vi "windowIcon.vi"(8 "Error In":errorcluster, 11 "LQGuiEngine In":refnum<class "LQGuiEngine.lvclass">) -> (0 "Error Out":errorcluster, 2 "Value":refnum<class "QIcon.lvclass">, 3 "LQGuiEngine Out":refnum<class "LQGuiEngine.lvclass">)   [LabVIEW 2014, in "LQGuiEngine.lvclass"]
doc: "LabVIEW-specific documentation is not yet available. See <b>http://doc.qt.io/qt-5/QGuiApplication.html#windowIcon</b>"
uses:
  LQGuiEngine.lvclass
  QIcon/QIcon.lvclass
  LQ Core/LQIdentity/LQIdentity.lvclass/LQIdentity.ctl
  LQ Core/LQSerialData/LQSerialData.lvclass/LQSerialData.ctl
  LQ Core/LQ Core.lvlib
  LQ Core/LQIdentity/LQIdentity.lvclass
  LQ Core/LQSerialData/LQSerialData.lvclass
panel:
  # "Copyright (c) 2016 Sze Howe Koh\n\nThis Source Code Form is subject to the terms of the Mozilla Public\nLicense, v. 2.0. If a copy of the MPL was not distributed with this\nfile, You can obtain one at http://mozilla.org/MPL/2.0/."
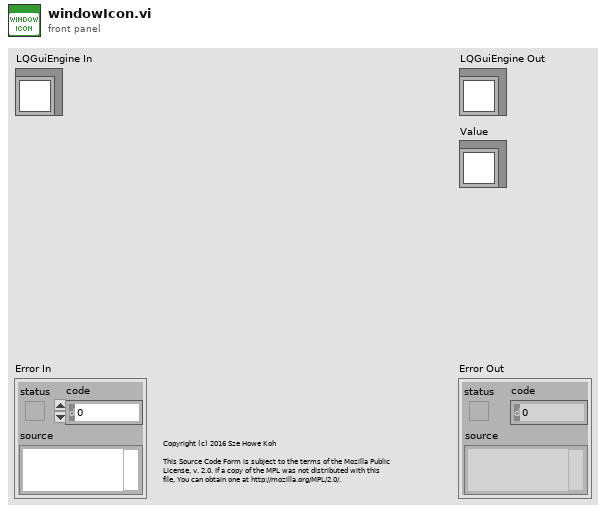
[diagram p1: front panel]
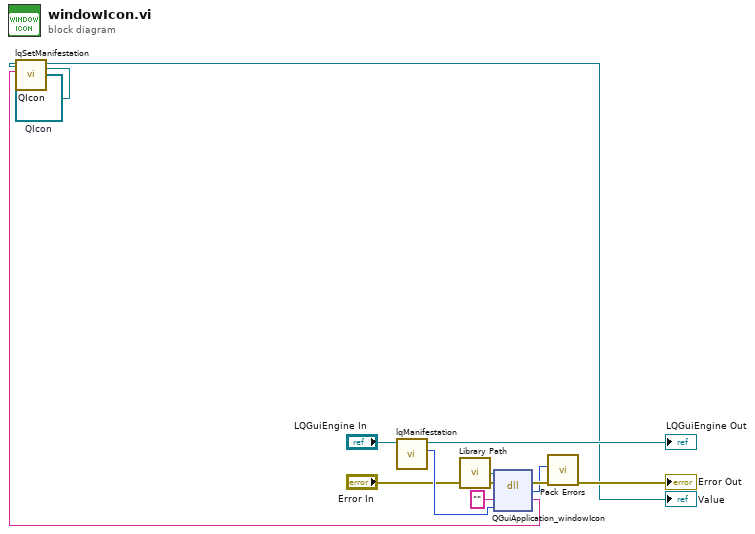
[diagram p0: block diagram]
diagram:
  w1 = refnum<class "QIcon.lvclass"> refnum  # QIcon
  n1 = call "lqManifestation.vi"("LQIdentity in"="LQGuiEngine In") -> ("Manifestation"=w8:u64, "LQIdentity out"=→"LQGuiEngine Out":refnum<class "LQGuiEngine.lvclass">)  [unwired: 9 in]
  n2 = call "Library Path.vi"() -> ("Library Path"=w9:path)
  n3 = dll-call lib="?" fn="QGuiApplication_windowIcon"(path in=w9, error in="Error In", "_retVal"="" ("retVal"), "_instance"=w8) -> (error out=w6:errorcluster, w4:i32, "_retVal"=w2:string)  [unwired: 2 in, 1 out]
  n4 = call "lqSetManifestation.vi"("Manifestation"=w2, "LQSerialData in"=w1) -> ("LQSerialData out"=→"Value":refnum<class "QIcon.lvclass">)  [unwired: 8 in, 1 out]
  n5 = call "Pack Errors.vi"("Error In"=w6, "Error Code"=w4) -> ("Error Out"=→"Error Out":errorcluster)  [unwired: 9 in]
